vi "Idle_Check_Timer.vi"(1 "Time Interval":T1=0.2 min=0.1 max=9999999.0, 2 "Previous Time In (Sec)":dbl) -> (4 "Idle?":bool, 6 "Previous Time Out (Sec)":dbl)   [LabVIEW 2020]
uses:
  Controls/Idle_Timer_disp.ctl
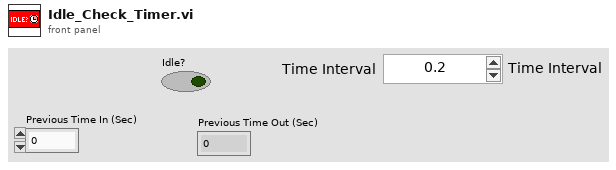
[diagram p1: front panel]
types:
  T1 = typedef "Idle_Timer_disp.ctl" = dbl
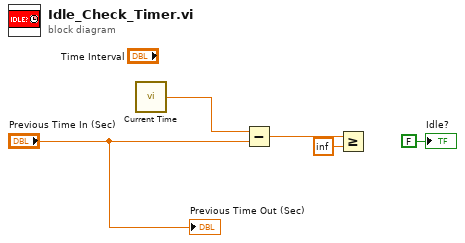
[diagram p0: block diagram]
diagram:
  n1 = call <userlib>:"Current Time.vi"() -> ("Current Time (Sec)"=w4:dbl)  [unwired: 15 in]
  n2 = Subtract(x=w4, y="Previous Time In (Sec)") -> (x-y=w5:dbl)
  n3 = Greater Or Equal?(x=w5, y=T1 inf ("Time Interval")) -> ()  [unwired: 1 out]
  "Idle?" <- FALSE ("Idle?")
  "Previous Time Out (Sec)" <- "Previous Time In (Sec)"
